vi "SearchForSubpanelsInDefault.vi"(8 "error in (no error)":errorcluster, 11 "SMO.UI.MAUI in":refnum<class "SMO.UI.MAUI.lvclass">) -> (0 "error out":errorcluster, 2 "Array":path[](array[path]), 3 "SMO.UI.MAUI out":refnum<class "SMO.UI.MAUI.lvclass">, 4 "Subpanels Found?":bool)   [LabVIEW 2020, in "SMO.UI.MAUI.lvclass"]
uses:
  SMO.UI.MAUI.lvclass
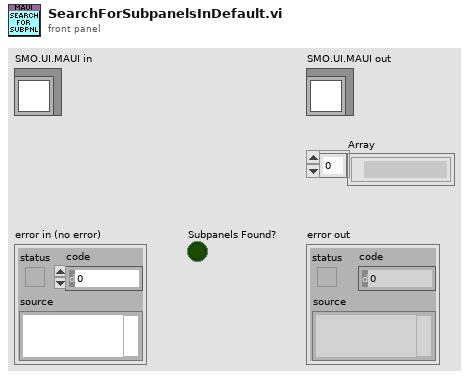
[diagram p1: front panel]
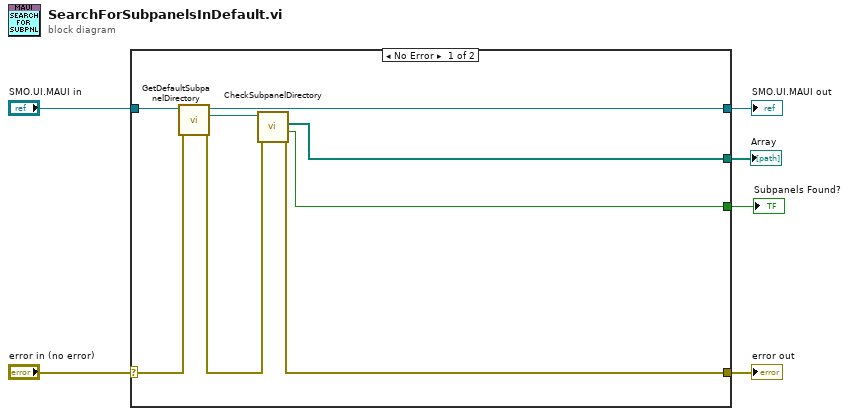
[diagram p0: block diagram]
diagram:
  n1 = case shown="No Error" "error in (no error)" {
    selector: "error in (no error)" -> [w14 w16]
    tunnel: [w9 w16] -> w5
    tunnel: [w13 w15] -> w3
    tunnel: "SMO.UI.MAUI in" -> [w12 w15]
    tunnel: [w8 _] -> w2
    tunnel: [w7 _] -> w1
    frame No Error {
      n2 = call "GetDefaultSubpanelDirectory.vi"("error in (no error)"=w14, "SMO.UI.MAUI in"=w12) -> ("error out"=w10:errorcluster, "Default Subpanel Directory"=w11:path, "SMO.UI.MAUI out"=w13:refnum<class "SMO.UI.MAUI.lvclass">)  [unwired: 7 in]
      n3 = call "CheckSubpanelDirectory.vi"("error in (no error)"=w10, "Path"=w11) -> ("error out"=w9:errorcluster, "Subpanels Found?"=w7:bool, "Array"=w8:path[])  [unwired: 6 in, 1 out]
    }
    frame Error {
    }
  }
  "error out" <- w5
  "SMO.UI.MAUI out" <- w3
  "Array" <- w2
  "Subpanels Found?" <- w1
